vi "miernik.vi"() -> ()   [LabVIEW 2018]
panel:
  out "napiêcie":dbl
  out "czestotliwoœæ":dbl
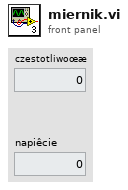
[diagram p1: front panel]
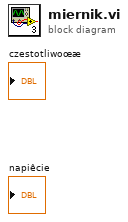
[diagram p0: block diagram]
diagram:
